vi "array with numeric addition.vi"() -> ()   [LabVIEW 2021]
panel:
  out "x+y":dbl[](array[numeric])
  in  "Numeric":dbl
  in  "Array":dbl[](array[numeric])
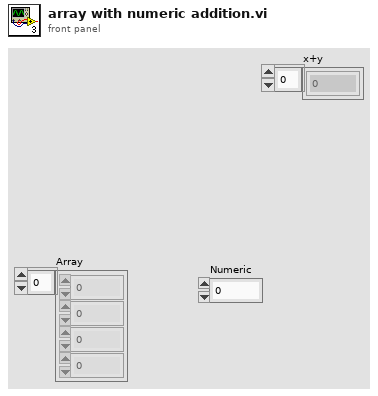
[diagram p1: front panel]
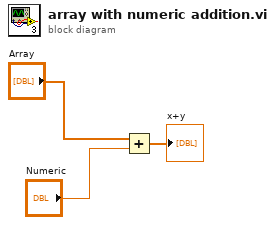
[diagram p0: block diagram]
diagram:
  n1 = Add(x="Array", y="Numeric") -> (x+y=→"x+y":dbl[])
